vi "remotecall.vi"() -> ()   [LabVIEW 2015]
panel:
  out "Numeric":i32
  out "Control Value:Get":variant
  in  "Fun":enum16{"Count", "Init"}(ring)
  in  "timeout ms (60000)":i32=60000
  in  "machine name (\"\":  open local reference)":string="127.0.0.1"
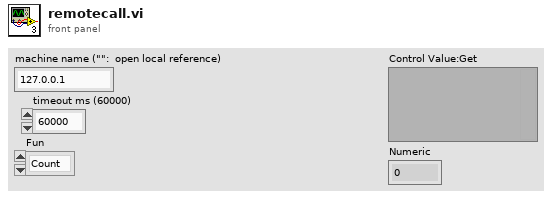
[diagram p1: front panel]
types:
  T1 = enum32{"Invalid", "Standard", "Closed", "Hidden", "Minimized", "Maximized"}
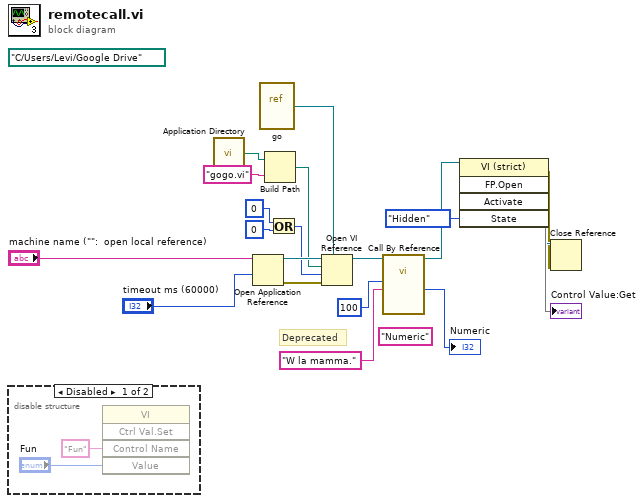
[diagram p0: block diagram]
diagram:
  (unwired) "Numeric" ("Control Name")
  (unwired) path "C:/Users/Levi/Google Drive" ("vi path")
  # "Deprecated"
  n1 = disable-structure shown="Disabled" {
    frame Disabled {
      n2 = invoke class="VI" method="Ctrl Val.Set"("Control Name"="Fun", "Value"="Fun") -> ()  [unwired: 3 in, 5 out]
    }
    frame Enabled {
    }
  }
  n3 = call <vilib>:"Application Directory.vi"() -> ("Application Directory"=w14:path)
  n4 = Open Application Reference(9:"timeout ms (60000)", 11:"machine name (\"\":  open local reference)") -> (0:w18:errorcluster, 3:w19:refnum<vi>)  [unwired: 2 in]
  n5 = vi-ref "go.vi"() -> (w7:refnum<vi>)
  n6 = Build Path(base path=w14, name or relative path="gogo.vi") -> (appended path=w15:path)
  n7 = Or(x=0 ("options"), y=0 ("options")) -> (x .or. y?=w11:i32)
  n8 = Open VI Reference(type specifier VI Refnum (for type only)=w7, application reference (local)=w19, vi path=w15, options=w11, error in (no error)=w18) -> (vi reference=w6:refnum<vi>)  [unwired: 1 in, 1 out]
  n9 = call-by-ref "?"(reference=w6, "string"="W la mamma.", "milliseconds to wait"=u32 100) -> (reference out=w5:refnum<vi>, "Numeric"=→"Numeric":i32)  [unwired: 10 in, 1 out]
  n10 = invoke class="VI (strict)" method="FP.Open"(reference=w5, "State"=T1."Hidden") -> (reference out=w9:refnum<vi>, error out=w8:errorcluster, "Open FP"=→"Control Value:Get")  [unwired: 3 in, 2 out]
  n11 = Close Reference(reference=w9, error in (no error)=w8) -> ()  [unwired: 1 out]
